vi "Read Settings.vi"(8 "error in":errorcluster, 11 "Controller in":refnum<class "Controller.lvclass">) -> (0 "error out":errorcluster, 2 "App Settings":T4 {"PLC Settings"."Sleep Address" format="%.0x"}, 3 "Controller out":refnum<class "Controller.lvclass">)   [LabVIEW 2022 SP3, in "Controller.lvlib" / "Controller.lvclass"]
uses:
  Controller.lvclass
  Typedefs/Storage Settings.ctl
  Typedefs/Image Formats.ctl
  Typedefs/PLC Settings.ctl
  Controller.lvclass/Controller.ctl
  <vilib>/Utility/config.llb/Read Key (U32).vi
  <vilib>/Utility/config.llb/Read Key (String).vi
  <vilib>/Utility/config.llb/Read Key (Path).vi
  <vilib>/Utility/config.llb/Read Key (Boolean).vi
  <vilib>/Utility/config.llb/NI_LVConfig.lvlib
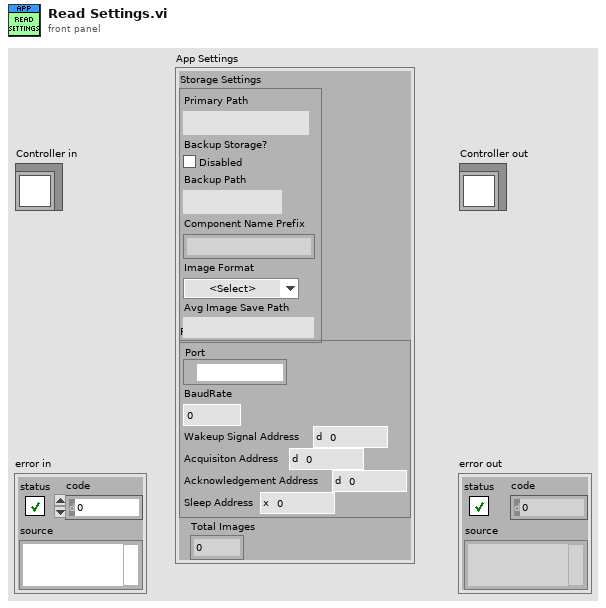
[diagram p1: front panel]
types:
  T1 = typedef "Storage Settings.ctl" = cluster{"Primary Path":path, "Backup Storage?":bool, "Backup Path":path, "Component Name Prefix":string, "Image Format":T2, "Avg Image Save Path":path}
  T2 = typedef "Image Formats.ctl" = enum16{"<Select>", "TIFF", "RAW"}
  T3 = typedef "PLC Settings.ctl" = cluster{"Port":refnum<visa-resource-name>, "BaudRate":u32, "Wakeup Signal Address ":u16, "Acquisiton Address":u16, "Acknowledgement Address":u16, "Sleep Address":u32}
  T4 = cluster{"Storage Settings":T1, "PLC Settings":T3, "Total Images":u32}
  T5 = cluster{"Config File ":path, "Configuration":path, "Event Log":path, "Error Log":path}
  T6 = typedef "NI_LVConfig.lvlib/Config Data RefNum.ctl" = refnum<k1>
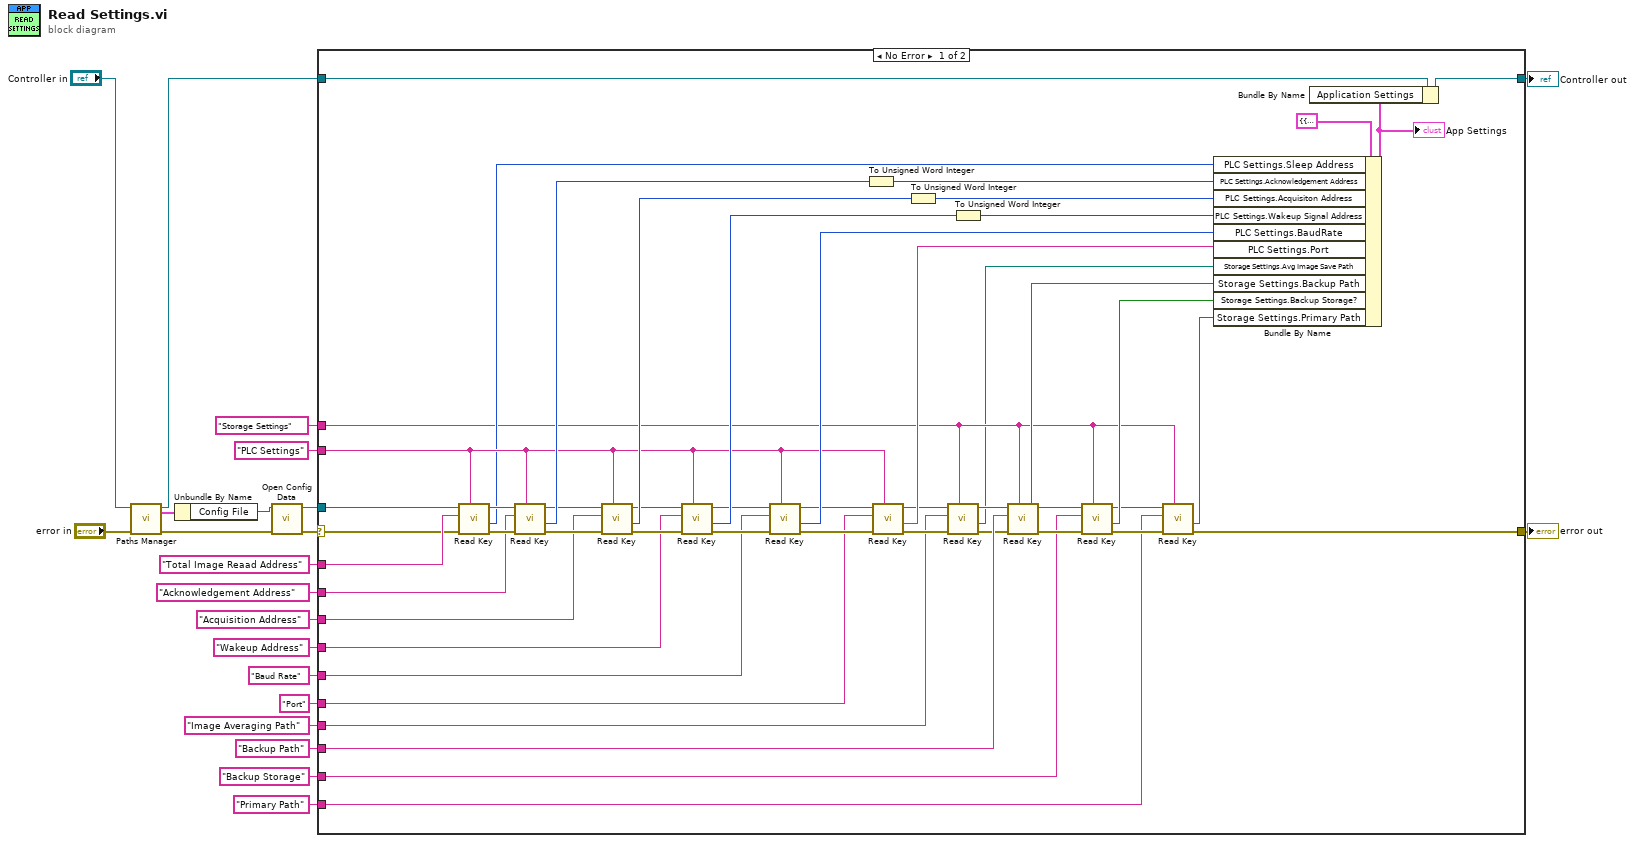
[diagram p0: block diagram]
diagram:
  n1 = call "Paths Manager.vi"("error in"="error in", "Controller in"="Controller in") -> ("error out"=w9:errorcluster, "Paths"=w6:T5, "Controller out"=w5:refnum<class "Controller.lvclass">)  [unwired: 7 in]
  n2 = Unbundle By Name(w6) -> ("Config File"=w4:path)
  n3 = call <vilib>:"Open Config Data.vi"("error in (no error)"=w9, "configuration file path"=w4) -> ("error out"=w8:errorcluster, "refnum"=w3:T6)  [unwired: 7 in, 1 out]
  n4 = case shown="No Error" w8 {
    selector: w8 -> [w32 w74]
    tunnel: [w64 w74] -> w21
    tunnel: [w39 w73] -> w2
    tunnel: w5 -> [w38 w73]
    tunnel: "Total Image Reaad Address" -> [w56 _]
    tunnel: "Acknowledgement Address" -> [w55 _]
    tunnel: "Acquisition Address" -> [w54 _]
    tunnel: "Wakeup Address" -> [w53 _]
    tunnel: "Baud Rate" -> [w52 _]
    tunnel: "Port" -> [w51 _]
    tunnel: "Backup Path" -> [w50 _]
    tunnel: "Backup Storage" -> [w49 _]
    tunnel: "Primary Path" -> [w48 _]
    tunnel: "Storage Settings" -> [w26 _]
    tunnel: "PLC Settings" -> [w40 _]
    tunnel: w3 -> [w31 _]
    tunnel: "Image Averaging Path" -> [w25 _]
    frame No Error {
      n5 = call-poly <vilib>:"Read Key.vi"("section"=w40, "error in (no error)"=w32, "key"=w56, "refnum"=w31) -> ("error out"=w67:errorcluster, "value"=w33:u32, "refnum out"=w47:T6)  [unwired: 4 in, 1 out]
      n6 = call-poly <vilib>:"Read Key.vi"("section"=w40, "error in (no error)"=w67, "key"=w55, "refnum"=w47) -> ("error out"=w71:errorcluster, "value"=w63:u32, "refnum out"=w46:T6)  [unwired: 4 in, 1 out]
      n7 = call-poly <vilib>:"Read Key.vi"("section"=w40, "error in (no error)"=w71, "key"=w54, "refnum"=w46) -> ("error out"=w66:errorcluster, "value"=w62:u32, "refnum out"=w45:T6)  [unwired: 4 in, 1 out]
      n8 = call-poly <vilib>:"Read Key.vi"("section"=w40, "error in (no error)"=w66, "key"=w53, "refnum"=w45) -> ("error out"=w68:errorcluster, "value"=w61:u32, "refnum out"=w44:T6)  [unwired: 4 in, 1 out]
      n9 = call-poly <vilib>:"Read Key.vi"("section"=w40, "error in (no error)"=w68, "key"=w52, "refnum"=w44) -> ("error out"=w65:errorcluster, "value"=w60:u32, "refnum out"=w43:T6)  [unwired: 4 in, 1 out]
      n10 = To Unsigned Word Integer(number=w63) -> (unsigned 16bit integer=w37:u16)
      n11 = call-poly <vilib>:"Read Key.vi"("section"=w40, "error in (no error)"=w65, "key"=w51, "refnum"=w43) -> ("error out"=w30:errorcluster, "value"=w34:string, "refnum out"=w28:T6)  [unwired: 4 in, 1 out]
      n12 = To Unsigned Word Integer(number=w62) -> (unsigned 16bit integer=w36:u16)
      n13 = call-poly <vilib>:"Read Key.vi"("section"=w26, "error in (no error)"=w30, "key"=w25, "refnum"=w28) -> ("error out"=w29:errorcluster, "value"=w24:path, "refnum out"=w27:T6)  [unwired: 4 in, 1 out]
      n14 = To Unsigned Word Integer(number=w61) -> (unsigned 16bit integer=w35:u16)
      n15 = call-poly <vilib>:"Read Key.vi"("section"=w26, "error in (no error)"=w29, "key"=w50, "refnum"=w27) -> ("error out"=w70:errorcluster, "value"=w59:path, "refnum out"=w42:T6)  [unwired: 4 in, 1 out]
      n16 = call-poly <vilib>:"Read Key.vi"("section"=w26, "error in (no error)"=w70, "key"=w49, "refnum"=w42) -> ("error out"=w69:errorcluster, "value"=w58:bool, "refnum out"=w41:T6)  [unwired: 4 in, 1 out]
      n17 = call-poly <vilib>:"Read Key.vi"("section"=w26, "error in (no error)"=w69, "key"=w48, "refnum"=w41) -> ("error out"=w64:errorcluster, "value"=w57:path)  [unwired: 4 in, 2 out]
      n18 = Bundle By Name(cluster=T4 {"Storage Settings"={"Primary Path"=path "", "Backup Storage?"=FALSE, "Backup Path"=path "", "Component Name Prefix"="", "Image Format"=enum."<Select>", "Avg Image Save Path"=path ""}, "PLC Settings"={"Port"="", "BaudRate"=0, "Wakeup Signal Address "=0, "Acquisiton Address"=0, "Acknowledgement Address"=0, "Sleep Address"=0}, "Total Images"=0} ("Application Settings"), "PLC Settings.Sleep Address"=w33, "PLC Settings.Acknowledgement Address"=w37, "PLC Settings.Acquisiton Address"=w36, "PLC Settings.Wakeup Signal Address"=w35, "PLC Settings.BaudRate"=w60, "PLC Settings.Port"=w34, "Storage Settings.Avg Image Save Path"=w24, "Storage Settings.Backup Path"=w59, "Storage Settings.Backup Storage?"=w58, "Storage Settings.Primary Path"=w57) -> (w23:T4)
      "App Settings" <- w23
      n19 = Bundle By Name(cluster=w38, "Application Settings"=w23) -> (w39:refnum<class "Controller.lvclass">)
    }
    frame Error {
    }
  }
  "error out" <- w21
  "Controller out" <- w2
